vi "Create ADS Client.vi"(8 "error in (no error)":errorcluster, 11 "TwinCAT ADS in":refnum<class "TwinCAT ADS.lvclass">) -> (0 "error out":errorcluster, 3 "TwinCAT ADS out":refnum<class "TwinCAT ADS.lvclass">)   [LabVIEW 2018, in "TwinCAT ADS.lvclass"]
uses:
  TwinCAT ADS.lvclass
  TwinCAT.Ads
  TwinCAT ADS.lvclass/TwinCAT ADS.ctl
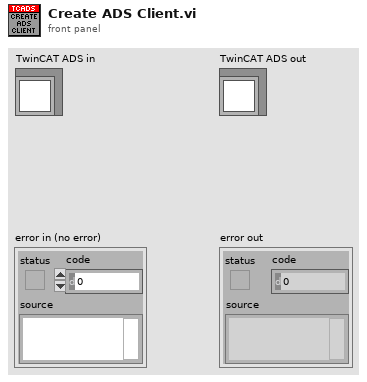
[diagram p1: front panel]
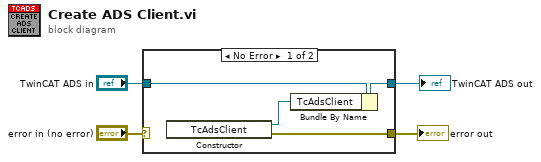
[diagram p0: block diagram]
diagram:
  n1 = case shown="No Error" "error in (no error)" {
    selector: "error in (no error)" -> [_ w10]
    tunnel: [w6 w10] -> w3
    tunnel: [w7 w9] -> w1
    tunnel: "TwinCAT ADS in" -> [w8 w9]
    frame No Error {
      n2 = constructor class="TcAdsClient"() -> (reference out=w5:refnum<k24>, error out=w6:errorcluster)  [unwired: 3 in, 1 out]
      n3 = Bundle By Name(cluster=w8, "TcAdsClient"=w5) -> (w7:refnum<class "TwinCAT ADS.lvclass">)
    }
    frame Error {
    }
  }
  "error out" <- w3
  "TwinCAT ADS out" <- w1
